vi "Read.vi"(8 "error in (no error)":errorcluster, 9 "Timeout ms (-1)":i32=-1, 11 "App ID in":u16) -> (0 "error out":errorcluster, 1 "Timed Out?":bool, 2 "Packet Data out":string, 3 "App ID out":u16, 4 "Exit?":bool)   [LabVIEW 2018, in "TCPServer.lvlib"]
uses:
  TCPServer.lvlib
  <vilib>/ErrorRing/Error Ring.xnode
  <vilib>/Utility/error.llb/Error Cluster From Error Code.vi
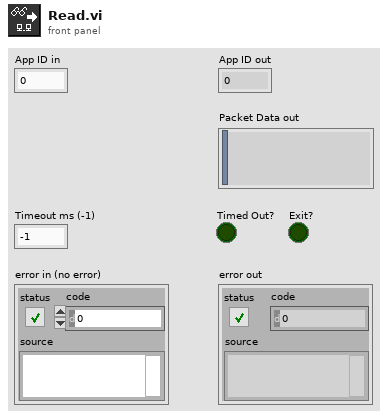
[diagram p1: front panel]
types:
  T1 = typedef "TCPServer.lvlib/App.ctl" = cluster{"Stack":refnum<queue>, "Cmd":cluster{"Conn":refnum<data-value>, "Daemon":refnum<vi>, "Counter":refnum<data-value>}, "Tlm":cluster{"Conn":refnum<data-value>, "Daemon":refnum<vi>, "Counter":refnum<data-value>}}
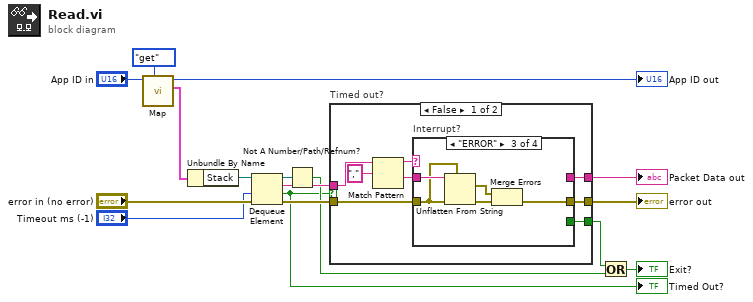
[diagram p0: block diagram]
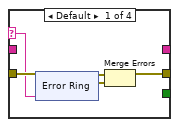
[diagram p2: hidden frame]
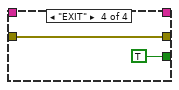
[diagram p4: hidden frame]
diagram:
  n1 = call "Map.vi"("Action"=enum8{"noop", "get", "set", "pop"}."get", "App ID in"="App ID in") -> ("App out"=w7:T1, "App ID out"=→"App ID out":u16)  [unwired: 7 in, 1 out]
  n2 = Unbundle By Name(w7) -> ("Stack"=w6:refnum<queue>)
  n3 = Dequeue Element(queue=w6, timeout in ms (-1)="Timeout ms (-1)", error in (no error)="error in (no error)") -> (queue out=w5:refnum<queue>, element=w14:string, timed out?=w1:bool, error out=w13:errorcluster)
  "Timed Out?" <- w1
  n4 = Not A Number/Path/Refnum?(number/path/refnum=w5) -> (NaN/Path/Refnum?=w4:bool)
  n5 = case "Timed out?" shown="False" w1 {
    tunnel: w14 -> [w24 _]
    tunnel: w13 -> [w22 w45]
    tunnel: [w19 w45] -> w12
    tunnel: [w18 _] -> w11
    tunnel: [w17 _] -> w2
    frame False {
      n6 = Match Pattern(string=w24, regular expression=",") -> (before substring=w21:string, after substring=w20:string)  [unwired: 1 in, 2 out]
      n7 = case "Interrupt?" shown="\"ERROR\"" w21 {
        selector: w21 -> [w25 _ _ _]
        tunnel: w22 -> [w26 w37 w40 w44]
        tunnel: w20 -> [_ w36 w41 _]
        tunnel: [w27 w37 w39 w44] -> w19
        tunnel: [_ w36 _ _] -> w18
        tunnel: [_ _ _ TRUE] -> w17
        frame Default {
          n8 = xnode "Error Ring"("parameter 0"=w25) -> ("error out"=w28:errorcluster)
          n9 = Merge Errors(w26, w28) -> (w27:errorcluster)
        }
        frame "CMD" {
        }
        frame "ERROR" {
          n10 = Unflatten From String(type=w40, binary string=w41, error in (no error)=w40) -> (value=w38:errorcluster, error out=w42:errorcluster)  [unwired: 2 in, 1 out]
          n11 = Merge Errors(w38, w42) -> (w39:errorcluster)
        }
        frame "EXIT" {
        }
      }
    }
    frame True {
    }
  }
  "error out" <- w12
  "Packet Data out" <- w11
  n12 = Or(x=w2, y=w4) -> (x .or. y?=→"Exit?":bool)
